vi "Reference Circle.vi"(9 "Radius":dbl, 10 "Frequency":dbl, 11 "Time":dbl) -> (3 "Reference Position":dbl[](array[numeric]))   [LabVIEW 2021]
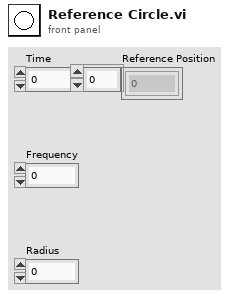
[diagram p1: front panel]
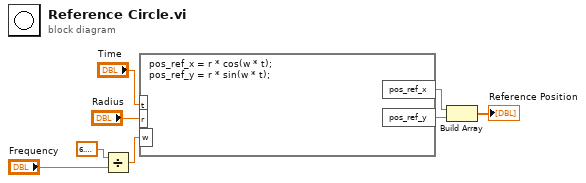
[diagram p0: block diagram]
diagram:
  n1 = Divide(x=6.283185307179586, y="Frequency") -> (x/y=w6:dbl)
  n2 = formula code="pos_ref_x = r * cos(w * t);\npos_ref_y = r * sin(w * t);"("t"="Time", "w"=w6, "r"="Radius") -> ("pos_ref_y"=w2:dbl, "pos_ref_x"=w3:dbl)
  n3 = Build Array(w3, w2) -> (→"Reference Position":dbl[])
